vi "Read piece info.vi"(11 "Piece in":refnum<class "Piece.lvclass">) -> (1 "Piece color":T1, 2 "Piece type":T2)   [LabVIEW 2015, in "Chesslib.lvlib" / "Piece.lvclass"]
uses:
  Piece.lvclass
  typedef/Piece type.ctl
  typedef/Color.ctl
  Piece.lvclass/Piece.ctl
  Chesslib.lvlib
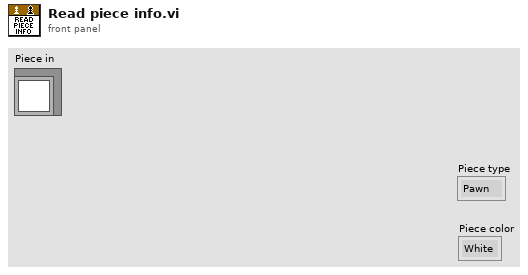
[diagram p1: front panel]
types:
  T1 = typedef "Chesslib.lvlib/Color.ctl" = enum16{"White", "Black"}
  T2 = typedef "Chesslib.lvlib/Piece type.ctl" = enum16{"Pawn", "Bishop", "Knight", "Rook", "Queen", "King"}
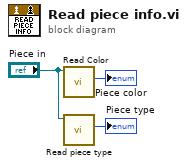
[diagram p0: block diagram]
diagram:
  n1 = call "Read Color.vi"("Piece in"="Piece in") -> ("Color"=→"Piece color":T1)  [unwired: 10 in]
  n2 = call-dynamic "Read piece type.vi"("Piece in"="Piece in") -> ("Piece type"=→"Piece type":T2)  [unwired: 10 in]
